vi "Finish Logging.vi"(0 "error in":errorcluster) -> (1 "error out":errorcluster, 2 "Extra Elements":i32)   [LabVIEW 2016]
uses:
  Refname/Queues.ctl
  Refname/Sensors.ctl
  Refname/Refname to String (Sensors).vi
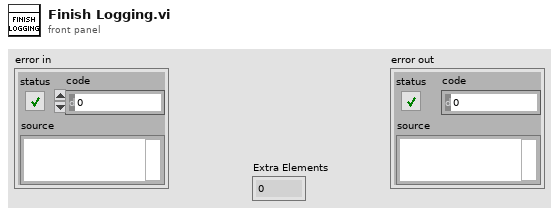
[diagram p1: front panel]
types:
  T1 = typedef "Sensors.ctl" = enum16{"DIP 1", "DIP 2", "DIP 3", "DIP 4", "IMU", "HuskieBoard"}
  T2 = typedef "Queues.ctl" = enum16{"Log Queue"}
  T3 = typedef "WPI_SerialPortRef.ctl" = cluster{"DevStatus":errorcluster, "Serial Port Name":refnum<visa-resource-name>}
  T4 = cluster{"Extra String":string, "Extra Data Exists":bool}
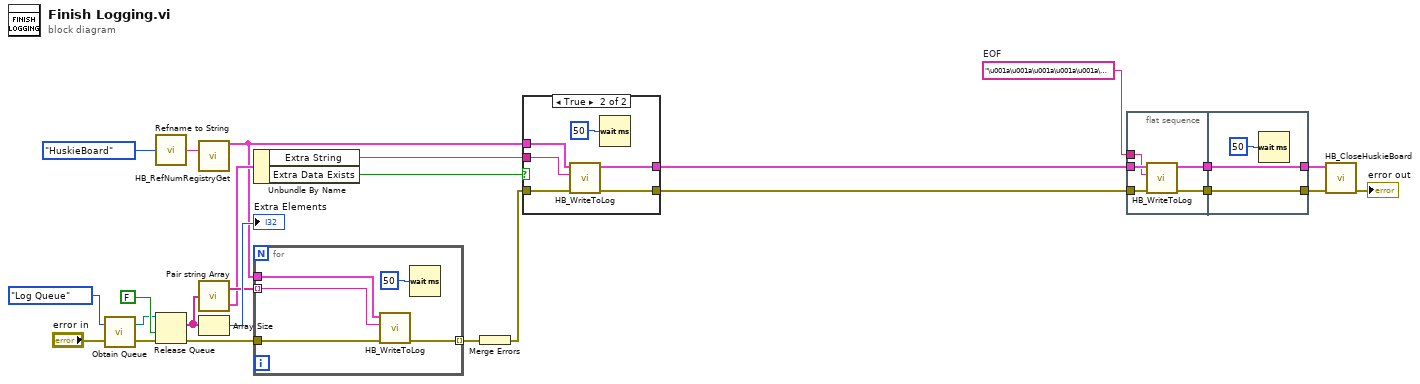
[diagram p0: block diagram]
diagram:
  w5 = "\u001a\u001a\u001a\u001a\u001a\u001a\u001a\u001a"  # EOF
  n1 = call "Obtain Queue.vi"("error in"="error in", "Queue"=Queues."Log Queue") -> ("error out"=w22:errorcluster, "Queue Ref"=w21:refnum<queue>)
  n2 = call-poly "Refname to String.vi"("Enum"=Sensors."HuskieBoard") -> ("String"=w19:string)
  n3 = Release Queue(queue=w21, force destroy? (F)=FALSE, error in (no error)=w22) -> (remaining elements=w15:string[], error out=w23:errorcluster)  [unwired: 1 out]
  n4 = call <vilib>:"HB_RefNumRegistryGet.vi"("refnum name"=w19) -> ("HBDevRef"=w12:T3)  [unwired: 13 in, 1 out]
  n5 = call "Pair string Array.vi"("Flat Array"=w15) -> ("Concatenated Strings"=w16:string[], "Extra Data"=w14:T4)
  n6 = Array Size(array=w15) -> (size(s)=→"Extra Elements":i32)
  n7 = Unbundle By Name(w14) -> ("Extra String"=w11:string, "Extra Data Exists"=w13:bool)
  n8 = for {
    tunnel: w16 -> [w30] mode=indexing
    tunnel: w23 -> [w29]
    tunnel: [w28] -> w17 mode=indexing
    tunnel: w12 -> [w27]
    n9 = call <vilib>:"HB_WriteToLog.vi"("error in (no error)"=w29, "Log string"=w30, "HBDevRef"=w27) -> ("error out"=w28:errorcluster)  [unwired: 7 in, 1 out]
    n10 = Wait (ms)(milliseconds to wait=u32 50) -> ()  [unwired: 1 out]
  }
  n11 = Merge Errors(w17) -> (w10:errorcluster)
  n12 = case shown="True" w13 {
    tunnel: w12 -> [w31 w38]
    tunnel: w11 -> [_ w37]
    tunnel: [w32 w36] -> w6
    tunnel: [w31 w35] -> w7
    tunnel: w10 -> [w32 w34]
    frame False {
    }
    frame True {
      n13 = call <vilib>:"HB_WriteToLog.vi"("error in (no error)"=w34, "Log string"=w37, "HBDevRef"=w38) -> ("error out"=w36:errorcluster, "HBDevRef"=w35:T3)  [unwired: 7 in]
      n14 = Wait (ms)(milliseconds to wait=u32 50) -> ()  [unwired: 1 out]
    }
  }
  n15 = flat-sequence {
    tunnel: w7 -> [w43]
    tunnel: w6 -> [w42]
    tunnel: w5 -> [w41]
    tunnel: [w40] -> w3
    tunnel: [w39] -> w2
    tunnel: [w45] -> w4
    tunnel: w3 -> [w45]
    tunnel: [w44] -> w1
    tunnel: w2 -> [w44]
    frame #0 {
      n16 = call <vilib>:"HB_WriteToLog.vi"("error in (no error)"=w42, "Log string"=w41, "HBDevRef"=w43) -> ("error out"=w39:errorcluster, "HBDevRef"=w40:T3)  [unwired: 7 in]
    }
    frame #1 {
      n17 = Wait (ms)(milliseconds to wait=u32 50) -> ()  [unwired: 1 out]
    }
  }
  n18 = call <vilib>:"HB_CloseHuskieBoard.vi"("error in (no error)"=w1, "HBDeviceRef"=w4) -> ("error out"=→"error out":errorcluster)  [unwired: 9 in]
